vi "Delete File.vi"(8 "error in (no error)":errorcluster caption="错误输入（无错误）", 9 "recycle":i32(ring)=2 items=["DeletePermanently"=2, "SendToRecycleBin"=3], 10 "File Path":path, 11 "FileSystem 输入":refnum<class "FileSystem.lvclass"> caption="DNL_LabVIEW Object in") -> (0 "error out":errorcluster caption="错误输出", 3 "FileSystem 输出":refnum<class "FileSystem.lvclass"> caption="DNL_LabVIEW Object out")   [LabVIEW 2012, in "FileSystem.lvclass"]
uses:
  FileSystem.lvclass
  FileSystem.lvclass/FileSystem.ctl
  Microsoft.VisualBasic
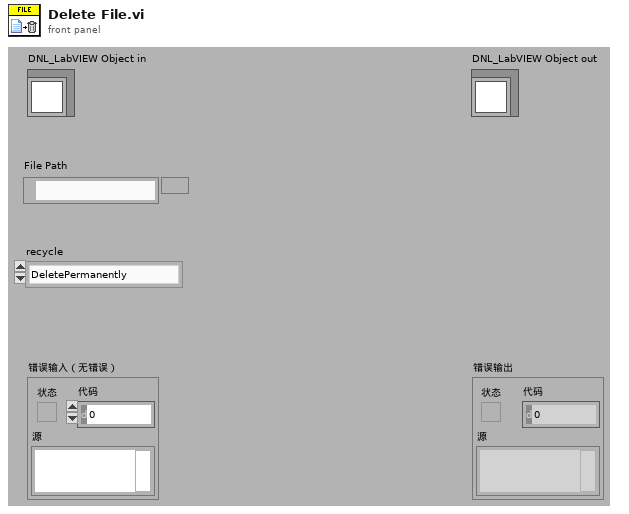
[diagram p1: front panel]
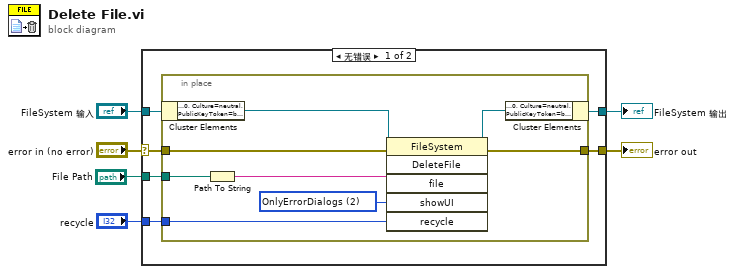
[diagram p0: block diagram]
diagram:
  n1 = case shown="无错误" "error in (no error)" {
    selector: "error in (no error)" -> [w10 w22]
    tunnel: [w9 w22] -> w5
    tunnel: [w11 w21] -> w3
    tunnel: "FileSystem 输入" -> [w12 w21]
    tunnel: "recycle" -> [w8 _]
    tunnel: "File Path" -> [w7 _]
    frame No Error {
      n2 = in-place {
        in-place-border: w10 -> [w18]
        in-place-border: [w17] -> w9
        in-place-border: w8 -> [w15]
        in-place-border: w7 -> [w14]
        w16 = 2 items=["OnlyErrorDialogs"=2, "AllDialogs"=3] ("showUI")
        n3 = in-place-cluster #1(w12) -> ("FileSystem"=w20:refnum<k24>)
        n4 = Path To String(path=w14) -> (string=w13:string)
        n5 = invoke class="FileSystem" method="DeleteFile"(reference=w20, error in=w18, "file"=w13, "showUI"=w16, "recycle"=w15) -> (reference out=w19:refnum<k24>, error out=w17:errorcluster)  [unwired: 1 in, 4 out]
        n6 = in-place-cluster #1("FileSystem"=w19) -> (w11:refnum<class "FileSystem.lvclass">)
      }
    }
    frame Error {
    }
  }
  "error out" <- w5
  "FileSystem 输出" <- w3
